vi "Init_Test.vi"(8 "error in (no error)":errorcluster caption="entrée d'erreur (pas d'erreur)", 11 "Wait_OpenFixture en entrée":refnum<class "Hide_Operator_Information.lvclass">) -> (0 "error out":errorcluster caption="sortie d'erreur", 3 "Wait_OpenFixture en sortie":refnum<class "Hide_Operator_Information.lvclass">)   [LabVIEW 2020, in "Library Test.lvlib" / "Hide_Operator_Information.lvclass"]
uses:
  Hide_Operator_Information.lvclass
  C:/Users/ngarcin/OneDrive - Altyor/Standard TB/Class/Test/Test (Default)/Test (Default).lvclass
  Commun VI/TypeDef/Commande Test/Commande Type Test.ctl
  Commun VI/TypeDef/Commande Test/Commande Value Type.ctl
  Test_Without_Instr/Test_Without_Inst.lvclass
  Instrument/Instrument (Default)/Class Instrument (Default).lvclass
  Hide_Operator_Information.lvclass/Hide_Operator_Information.ctl
  Commun VI/Library Commun.lvlib
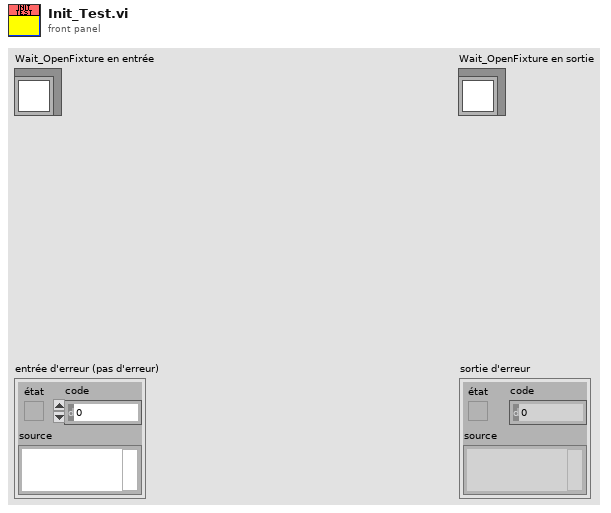
[diagram p1: front panel]
types:
  T1 = typedef "Library Commun.lvlib/Commande Value Type.ctl" = enum16{"None", "String", "Number", "Timestamp", "Boolean", "Array"}
  T2 = typedef "Library Commun.lvlib/Commande Type Test.ctl" = enum16{"Function", "Test", "Calculation"}
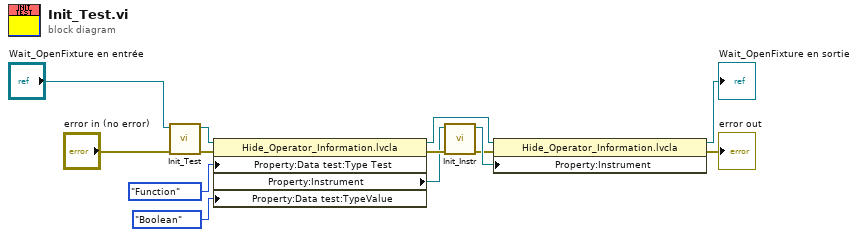
[diagram p0: block diagram]
diagram:
  n1 = call-parent "Init_Test.vi"("error in (no error)"="error in (no error)", "Test_Without_Inst en entrée"="Wait_OpenFixture en entrée") -> ("error out"=w10:errorcluster, "Test_Without_Inst en sortie"=w11:refnum<class "Hide_Operator_Information.lvclass">)  [unwired: 8 in]
  n2 = property class="Hide_Operator_Information.lvcla"(reference=w11, error in=w10, "Property:Data test:Type Test"=Commande_Type_Test."Function" ("Type Test"), "Property:Data test:TypeValue"=Commande_Value_Type."Boolean" ("TypeValue")) -> (reference out=w6:refnum<class "Hide_Operator_Information.lvclass">, error out=w8:errorcluster, "Property:Instrument"=w4:refnum<class "Class Instrument (Default).lvclass">)
  n3 = call-dynamic "Init_Instr.vi"("error in (no error)"=w8, "Class Instrument (Default) en entrée"=w4) -> ("error out"=w2:errorcluster, "Class Instrument (Default) en sortie"=w3:refnum<class "Class Instrument (Default).lvclass">)  [unwired: 8 in]
  n4 = property class="Hide_Operator_Information.lvcla"(reference=w6, error in=w2, "Property:Instrument"=w3) -> (reference out=→"Wait_OpenFixture en sortie":refnum<class "Hide_Operator_Information.lvclass">, error out=→"error out":errorcluster)
